vi "Write_new_group.vi"(8 "error in (no error)":errorcluster) -> (0 "error out":errorcluster, 3 "New Group":string)   [LabVIEW 2012]
uses:
  <vilib>/addons/database/NI_Database_API.lvlib
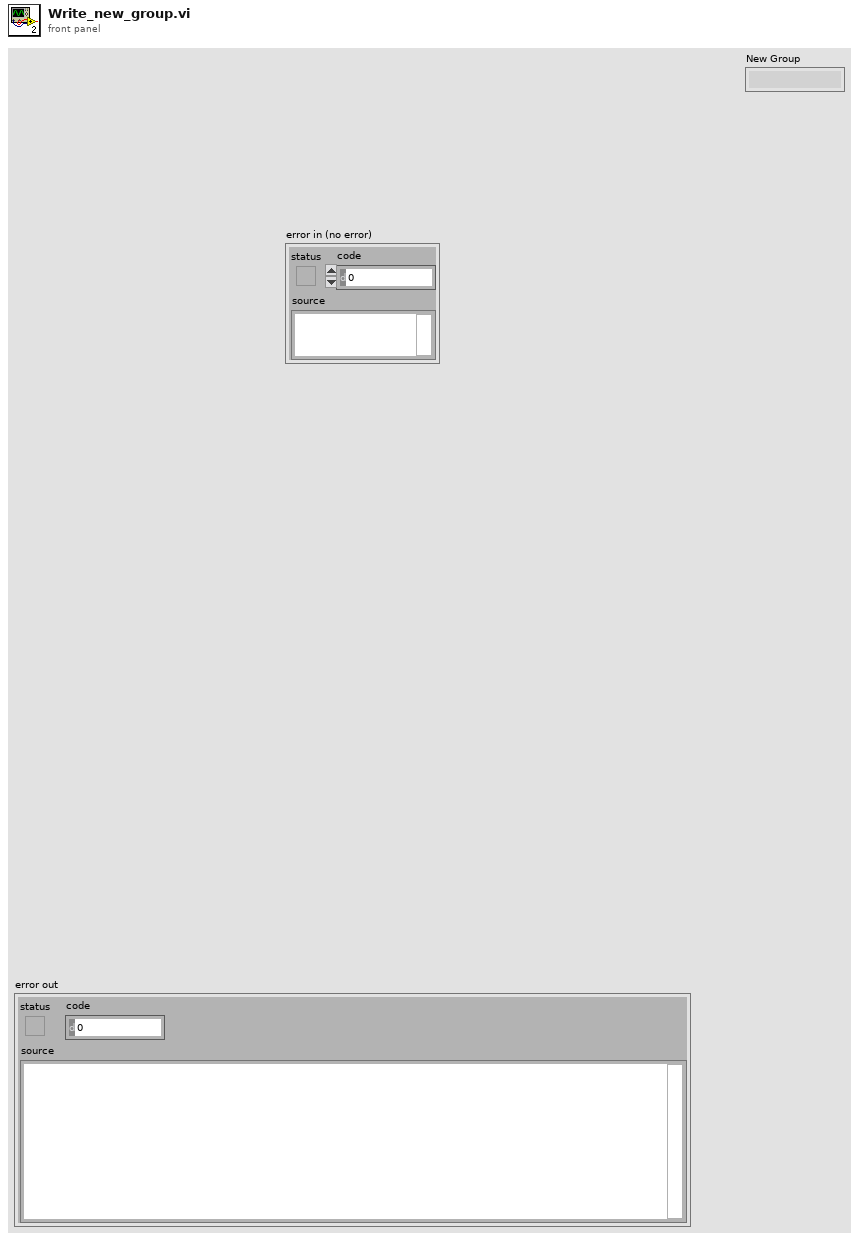
[diagram p1: front panel]
types:
  T1 = typedef "NI_Database_API.lvlib/Conn ObjectReference.ctl" = refnum<k1>
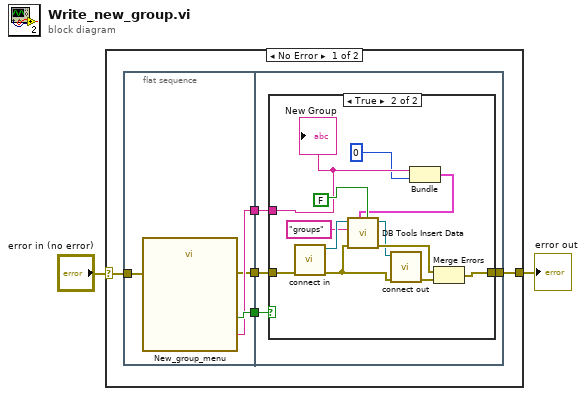
[diagram p0: block diagram]
diagram:
  n1 = case shown="No Error" "error in (no error)" {
    selector: "error in (no error)" -> [w7 w29]
    tunnel: [w6 w29] -> w1
    frame No Error {
      n2 = flat-sequence {
        tunnel: w7 -> [w9]
        tunnel: [w11] -> w5
        tunnel: [w8] -> w4
        tunnel: [w10] -> w3
        tunnel: [w15] -> w6
        tunnel: w5 -> [w14]
        tunnel: w4 -> [w13]
        tunnel: w3 -> [w12]
        frame #0 {
          n3 = call "New_group_menu.vi"("error in (no error)"=w9) -> ("Please Enter New Group"=w10:string, "Add new group"=w11:bool, "error out"=w8:errorcluster)  [unwired: 16 in]
        }
        frame #1 {
          n4 = case shown="True" w14 {
            tunnel: [w16 w21] -> w15
            tunnel: w13 -> [w16 w20]
            tunnel: w12 -> [_ w18]
            frame False {
            }
            frame True {
              n5 = call "connect in.vi"("error in (no error)"=w20) -> ("error out"=w27:errorcluster, "Database Connection"=w23:T1)  [unwired: 6 in, 1 out]
              n6 = Bundle("Please Enter New Group"=w18, 0) -> (w19:cluster{"Please Enter New Group":string, i32})  [unwired: 1 in]
              n7 = call <vilib>:"DB Tools Insert Data.vi"("create table? (F)"=FALSE, "data"=w19, "error in (no error)"=w27, "table"="groups", "connection reference"=w23) -> ("error out"=w26:errorcluster, "connection reference out"=w25:T1)  [unwired: 5 in]
              n8 = call "connect out.vi"("error in (no error)"=w27, "connection reference"=w25) -> ("error out"=w28:errorcluster)  [unwired: 9 in]
              n9 = Merge Errors(w26, w28) -> (w21:errorcluster)
              "New Group" <- w18
            }
          }
        }
      }
    }
    frame Error {
    }
  }
  "error out" <- w1
